vi "InterpolationAScan (SubVI).vi"(8 "Interpolation factor (n)":i32=1, 11 "magnitude":cluster{"f0":dbl, "df":dbl, "magnitude":dbl[]}) -> (3 "XY Graph":cluster{dbl[], dbl[]}(graph))   [LabVIEW 2017]
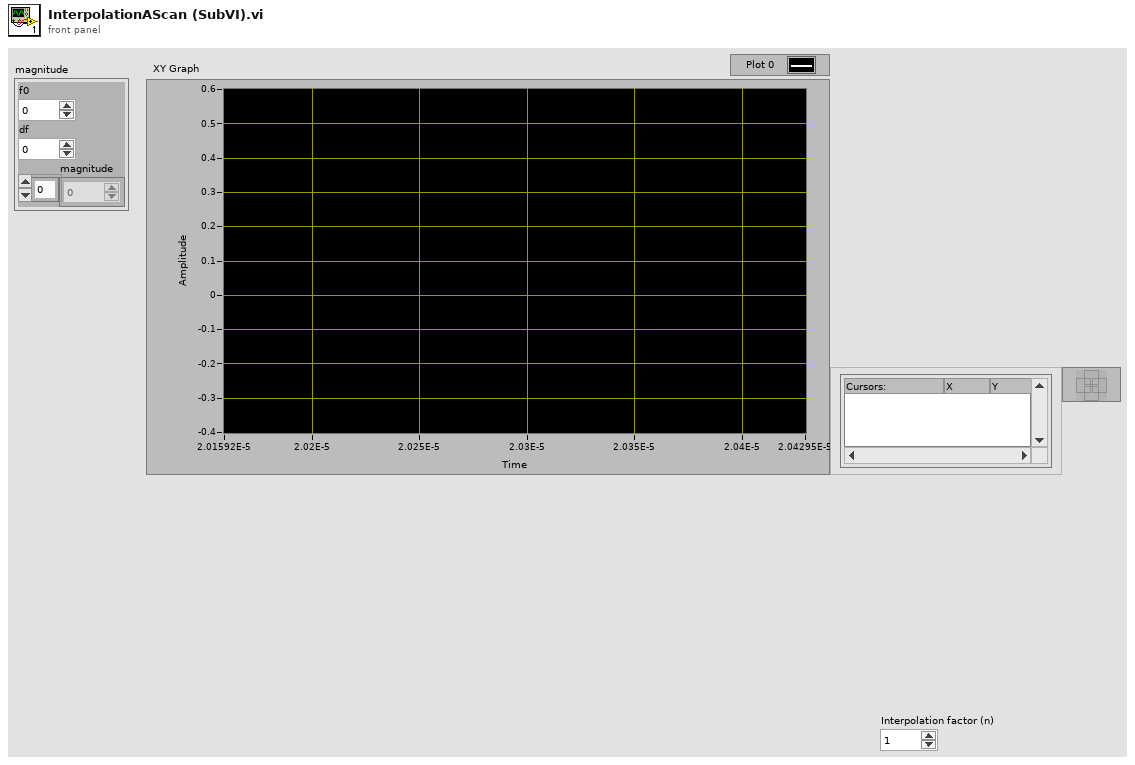
[diagram p1: front panel]
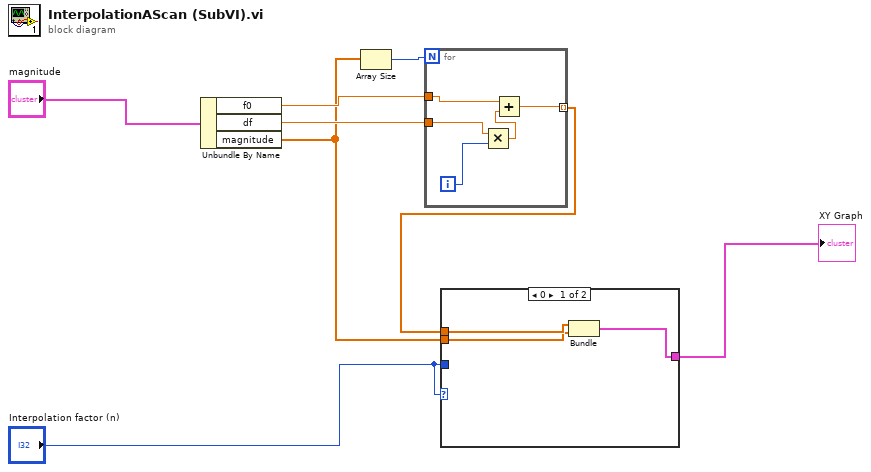
[diagram p0: block diagram]
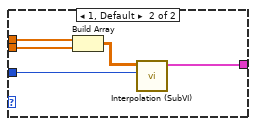
[diagram p2: hidden frame]
diagram:
  n1 = Unbundle By Name("magnitude") -> ("f0"=w7:dbl, "df"=w6:dbl, "magnitude"=w4:dbl[])
  n2 = Array Size(array=w4) -> (size(s)=w5:i32)
  n3 = for {
    N: w5 -> [_]
    tunnel: w7 -> [w13]
    tunnel: w6 -> [w11]
    tunnel: [w9] -> w3 mode=indexing
    i -> [w10]
    n4 = Multiply(x=w11, y=w10) -> (x*y=w12:dbl)
    n5 = Add(x=w13, y=w12) -> (x+y=w9:dbl)
  }
  n6 = case shown="0" "Interpolation factor (n)" {
    tunnel: "Interpolation factor (n)" -> [_ w21]
    tunnel: [w14 w20] -> w8
    tunnel: w4 -> [w15 w18]
    tunnel: w3 -> [w16 w17]
    frame 0 {
      n7 = Bundle(w16, "magnitude"=w15) -> (w14:cluster{dbl[], "magnitude":dbl[]})  [unwired: 1 in]
    }
    frame 1, Default {
      n8 = Build Array(w17, w18) -> (w19:dbl[][])
      n9 = call "Interpolation (SubVI).vi"("Interpolation factor (n)"=w21, "Original Data (X,Y)"=w19) -> ("Cluster"=w20:cluster{dbl[], dbl[]})  [unwired: 9 in]
    }
  }
  "XY Graph" <- w8
